vi "Tela Inicial.vi"() -> ()   [LabVIEW 2011]
doc: "VI que gerencia todas as opções e funções existentes na tela inicial do aplicativo."
panel:
  in  "HistoricodePartidas":bool
  in  "Sair":bool
  in  "Instruções":bool
  in  "Novo Jogo":bool
  # "Jogo da Velha"
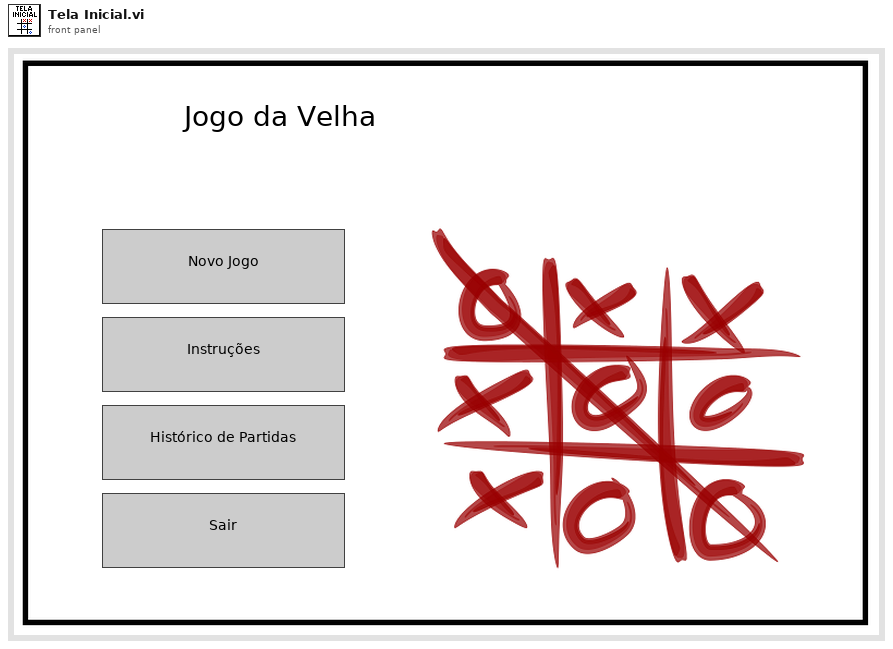
[diagram p1: front panel]
types:
  T1 = enum32{"invalid app kind", "Development System", "Run Time System", "Student Edition", "Embedded LabVIEW", "Evaluation", "Custom"}
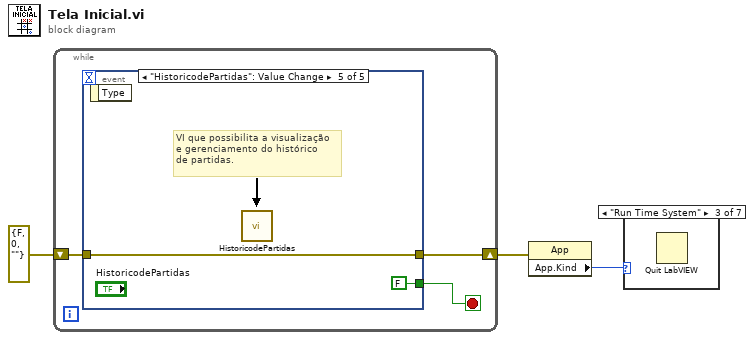
[diagram p0: block diagram]
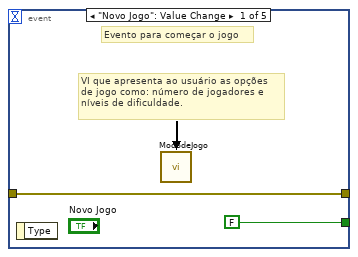
[diagram p8: hidden frame]
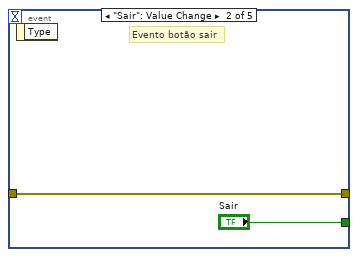
[diagram p9: hidden frame]
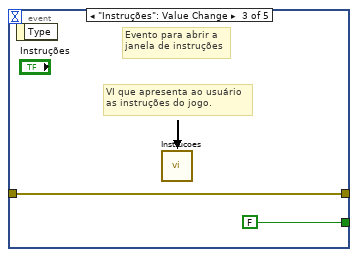
[diagram p10: hidden frame]
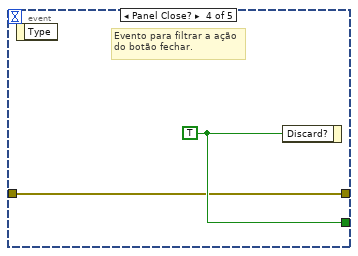
[diagram p11: hidden frame]
diagram:
  n1 = while {
    shift-right: [w4] -> w1
    shift-left: errorcluster {"status"=FALSE, "code"=0, "source"=""} ("error in (no error)") -> [w5]
    stop <- w6 stop-if-true
    n2 = event shown="[4] \"HistoricodePartidas\": Value Change" {
      selector: _ -> [_ _ _ _ _]
      dyn-events: _ -> [_ _ _ _ _]
      timeout: _ -> [_ _ _ _ _]
      tunnel: [FALSE "Sair" FALSE w14 FALSE ("Discard?")] -> w6
      tunnel: [w7 w9 w11 w13 w15] -> w4
      tunnel: w5 -> [w7 w9 w11 w13 w15]
      event "Novo Jogo": Value Change {
        # "VI que apresenta ao usuário as opções\nde jogo como: número de jogadores e\nníveis de dificuldade."
        # "Evento para começar o jogo"
        n3 = event-data() -> ()  [unwired: 1 in, 1 out]
        n4 = call "MododeJogo.vi"() -> ()  [unwired: 12 in]
      }
      event "Sair": Value Change {
        # "Evento botão sair"
        n5 = event-data() -> ()  [unwired: 1 in, 1 out]
      }
      event "Instruções": Value Change {
        # "VI que apresenta ao usuário\nas instruções do jogo."
        # "Evento para abrir a \njanela de instruções"
        n6 = event-data() -> ()  [unwired: 1 in, 1 out]
        n7 = call "Instrucoes.vi"() -> ()  [unwired: 12 in]
      }
      event Panel Close? {
        w14 = TRUE ("Discard?")
        # "Evento para filtrar a ação\ndo botão fechar."
        n8 = event-data() -> ()  [unwired: 1 in, 1 out]
        n9 = event-data("Discard?"=w14) -> ()  [unwired: 1 in, 1 out]
      }
      event "HistoricodePartidas": Value Change {
        # "VI que possibilita a visualização\ne gerenciamento do histórico \nde partidas."
        n10 = event-data() -> ()  [unwired: 1 in, 1 out]
        n11 = call "HistoricodePartidas.vi"() -> ()  [unwired: 12 in]
      }
    }
  }
  n12 = property class="App"(error in=w1) -> ("App.Kind"=w3:T1)  [unwired: 1 in, 2 out]
  n13 = case shown="\"Run Time System\"" w3 {
    frame "invalid app kind", Default {
    }
    frame "Development System" {
    }
    frame "Run Time System" {
      n14 = Quit LabVIEW() -> ()  [unwired: 1 in]
    }
    frame "Student Edition" {
    }
    frame "Embedded LabVIEW" {
    }
    frame "Evaluation" {
    }
    frame "Custom" {
    }
  }
